vi "process_display_IMAQ_imaq.vi"() -> ()   [LabVIEW 2011, in "Fiberscope_library.lvlib"]
uses:
  Fiberscope_library.lvlib
  typedefs/image_size_I32.ctl
  typedefs/control_process_state_enum.ctl
  typedefs/control_process_state_cluster.ctl
  typedefs/feedback_from_process_enum.ctl
  typedefs/feedback_to_watchdog.ctl
  <vilib>/Analysis/NI_AALBase.lvlib
  <vilib>/vision/Image Controls.llb/IMAQ Image.ctl
  typedefs/element_imaq_images_cluster.ctl
  typedefs/color_palette_enum.ctl
panel:
  in  "Ch1 lower":dbl
  in  "Ch0 lower":dbl
  in  "W2 Ch1 Color":T1=enum."Grayscale"
  in  "W2 Ch0 Color":T1=enum."Grayscale"
  in  "Ch1 upper":dbl
  in  "Ch0 upper":dbl
  out "Ch1 Max":dbl
  out "Ch0 Max":dbl
  in  "W1 Ch1 Color":T1=enum."Grayscale"
  out "Histogram Ch1":T2(graph)
  out "Histogram Ch0":T2(graph)
  out "Window 2":T3(plugin-control)
  out "Window 1":T3(plugin-control)
  in  "Ch1 Full range":bool
  in  "Ch1 Optimize":bool
  in  "W1 Ch0 Color":T1=enum."Grayscale"
  in  "Ch0 Full range":bool
  in  "Ch0 Optimize":bool
  out "Local exit":bool
  out "error out":errorcluster
  in  "error in":errorcluster
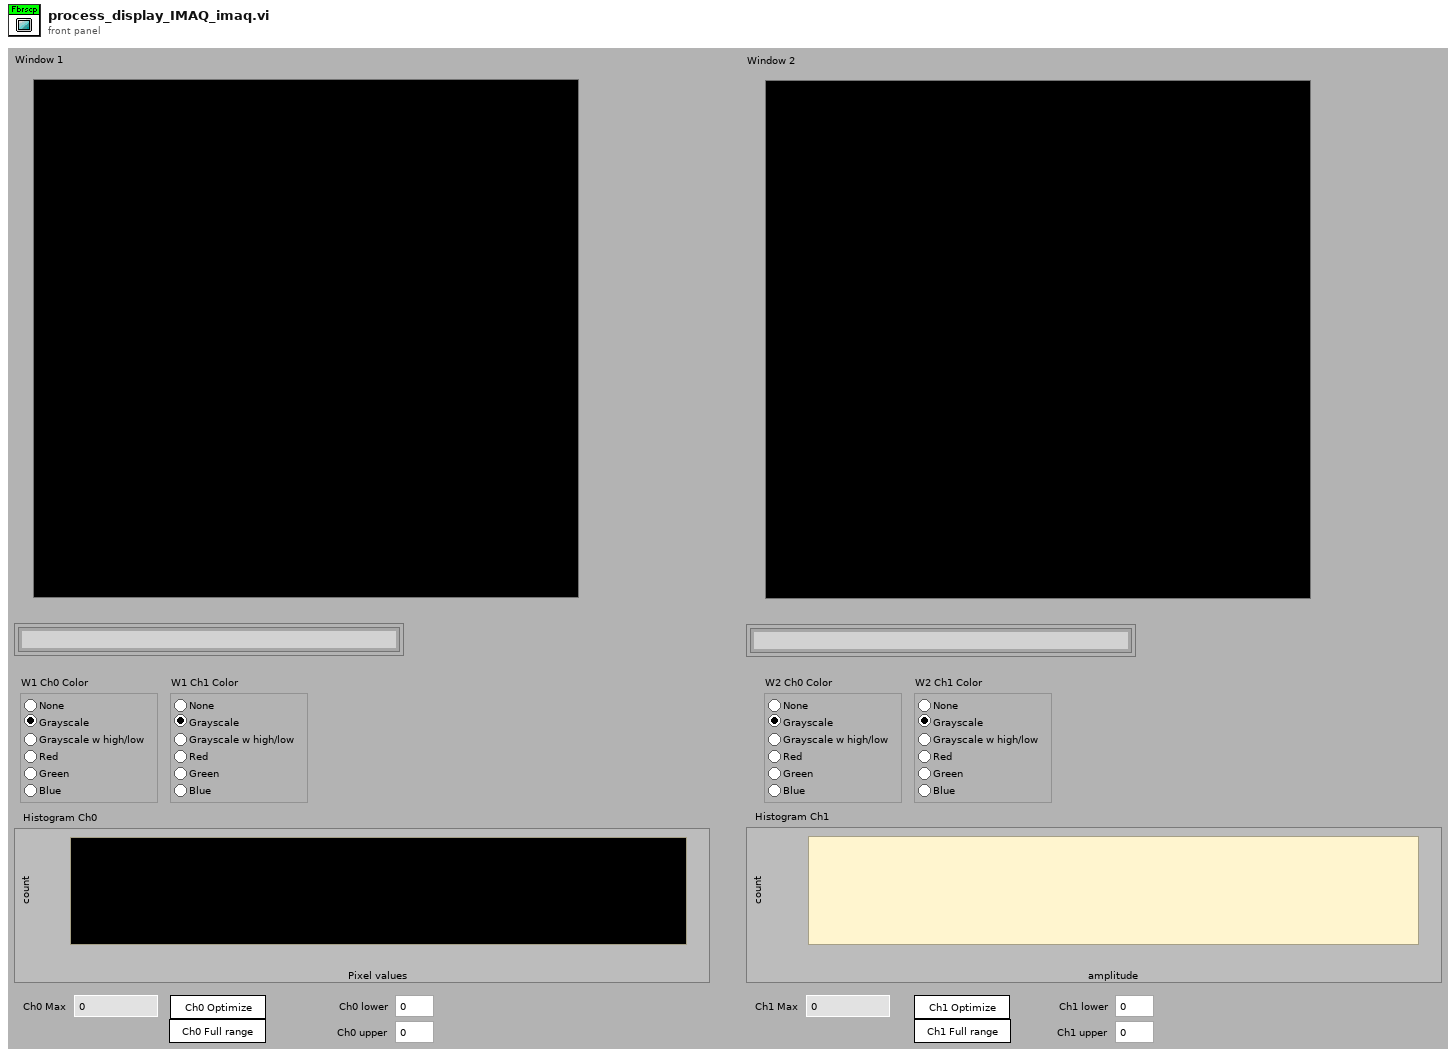
[diagram p1: front panel]
types:
  T1 = typedef "Fiberscope_library.lvlib/color_palette_enum.ctl" = enum32{"None", "Grayscale", "Grayscale w high/low", "Red", "Green", "Blue"}
  T2 = cluster{"X Values":dbl[], "Histogram: h(x)":i32[]}
  T3 = typedef "IMAQ Image.ctl" = refnum<image>
  T4 = typedef "Fiberscope_library.lvlib/element_imaq_images_cluster.ctl" = cluster{"Images":T3[], "#channels":i32, "Last element?":bool}
  T5 = typedef "Fiberscope_library.lvlib/feedback_to_watchdog.ctl" = cluster{"Feedback_from_process_enum":T6, "Process_name":string}
  T6 = typedef "Fiberscope_library.lvlib/feedback_from_process_enum.ctl" = enum16{"Has_initialised", "Changed_parameters", "Has_started", "Has_stopped", "Has_quitted", "Is_running", "Has_finished", "Custom"}
  T7 = typedef "Fiberscope_library.lvlib/control_process_state_cluster.ctl" = cluster{"Control_process_state_enum":T8, "variant":variant}
  T8 = typedef "Fiberscope_library.lvlib/control_process_state_enum.ctl" = enum16{"Init", "Quit", "Start", "Stop", "Change_parameters", "Running", "Finish", "Custom"}
  T9 = typedef "LVCursorListTypeDef.ctl" = cluster{"Name":string, "Color":u32, "Style":u8, "Point Style":u8, "Name Visible":bool, "Allow Drag":bool, "Cursor Mode":u32, "Plot":i32, "Index":i32, "Position":cluster{"X":dbl, "Y":dbl}, "X Scale":u32, "Y Scale":u32, "Watch Plots":i32[], "Watch All Plots":bool, "Plot Area":i32, "Label Offset":cluster{"X":dbl, "Y":dbl}}[]
  T10 = cluster{"Name":string, "Color":u32, "Style":u8, "Point Style":u8, "Name Visible":bool, "Allow Drag":bool, "Cursor Mode":u32, "Plot":i32, "Index":i32, "Position":cluster{"X":dbl, "Y":dbl}, "X Scale":u32, "Y Scale":u32, "Watch Plots":i32[], "Watch All Plots":bool, "Plot Area":i32, "Label Offset":cluster{"X":dbl, "Y":dbl}}
  T11 = typedef "Image Type" = u32
  T12 = typedef "Fiberscope_library.lvlib/image_size_I32.ctl" = i32
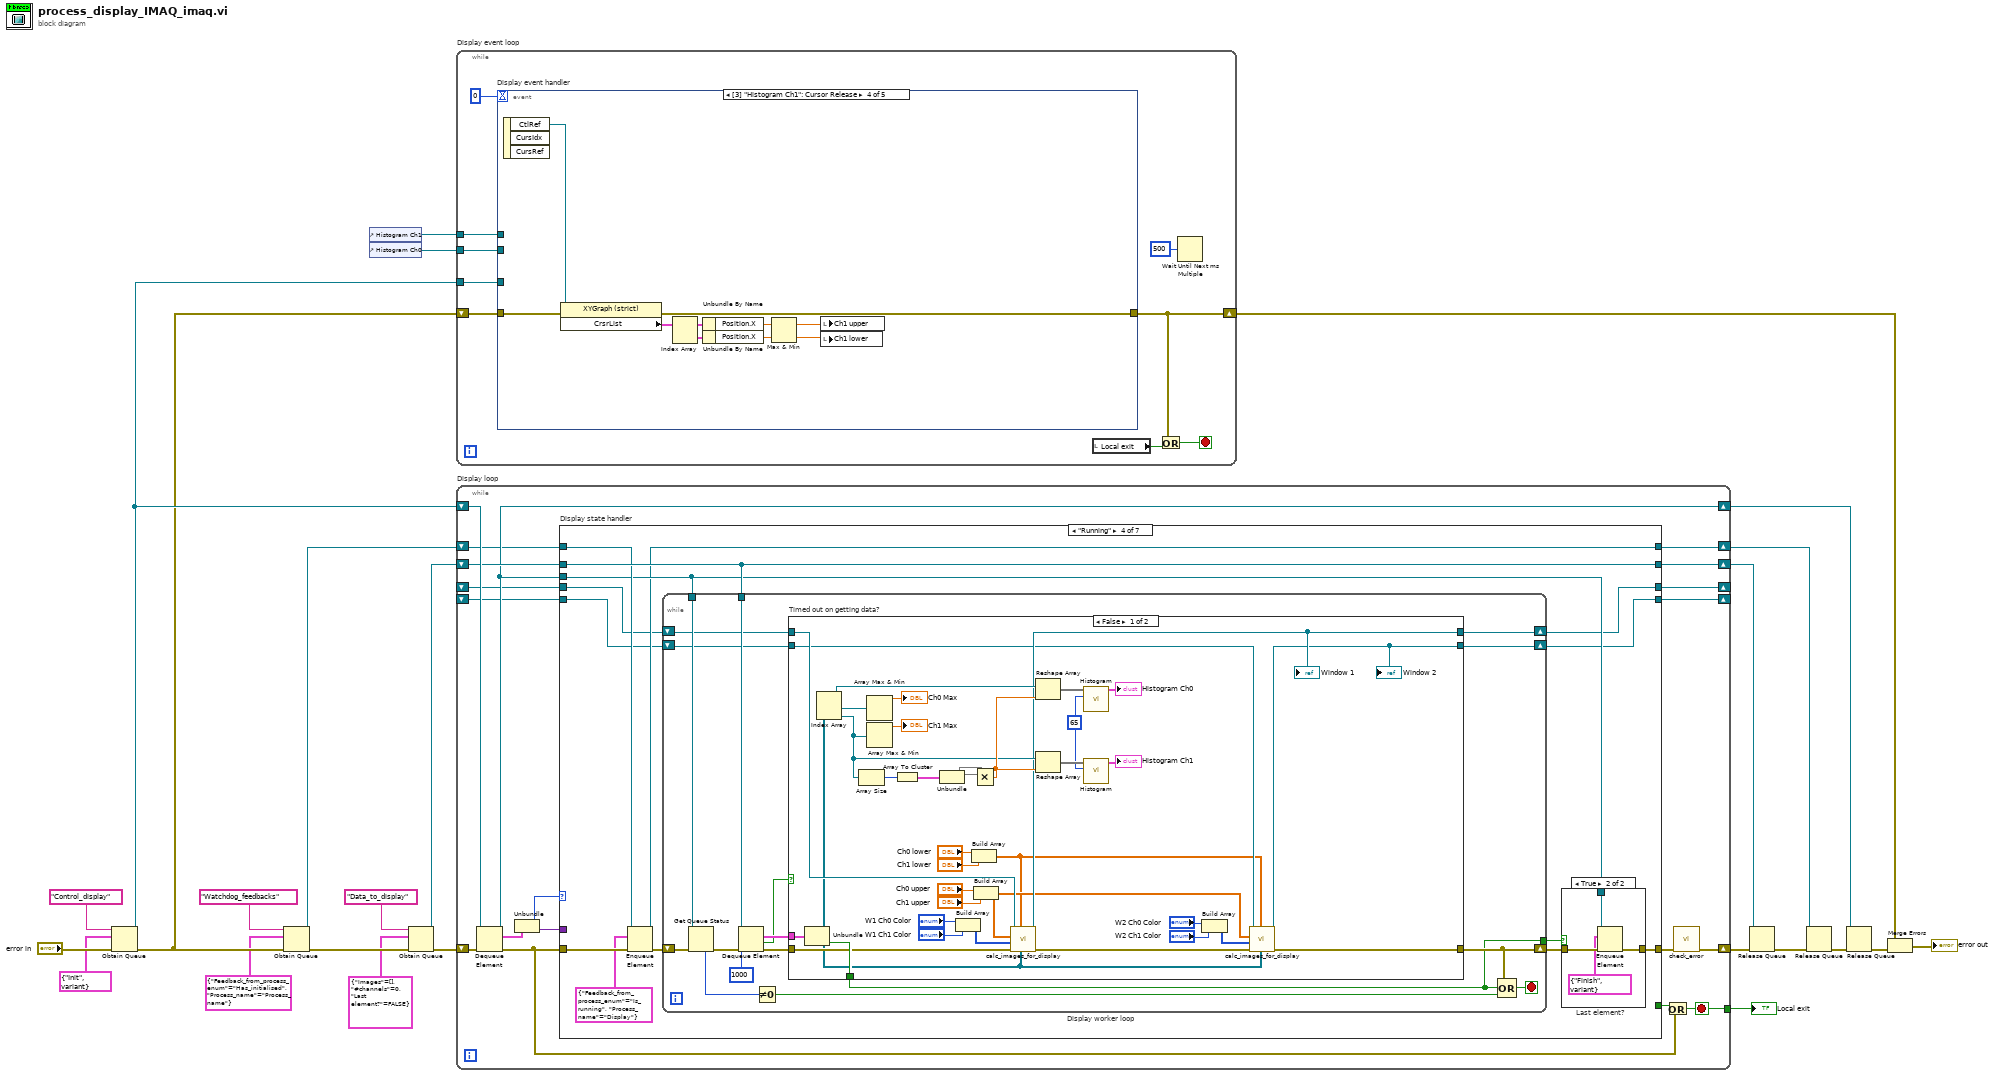
[diagram p0: block diagram]
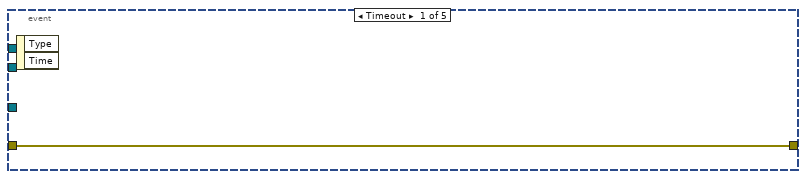
[diagram p2: hidden frame]
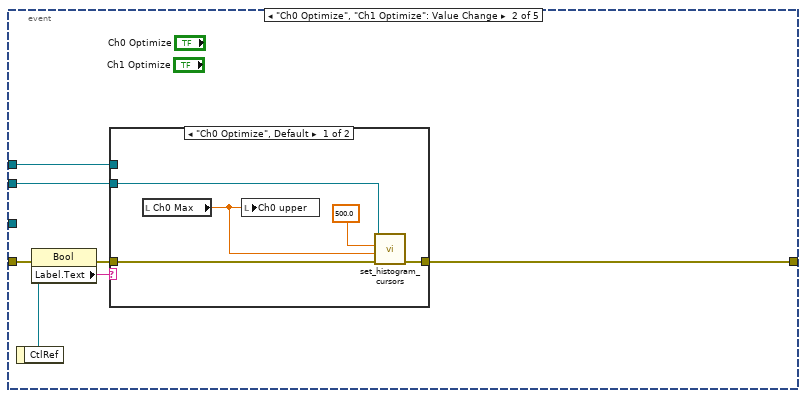
[diagram p3: hidden frame]
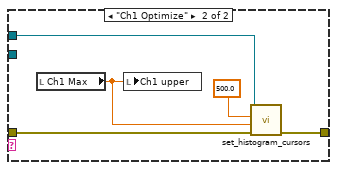
[diagram p4: hidden frame]
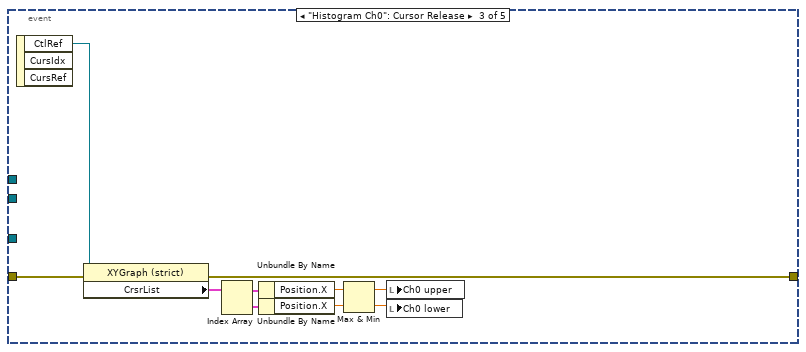
[diagram p5: hidden frame]
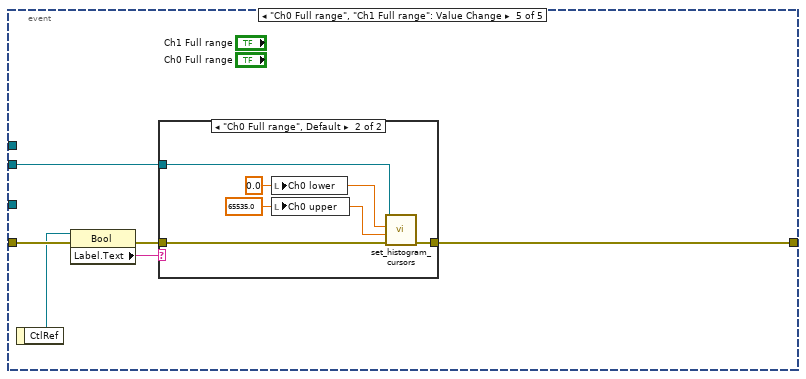
[diagram p6: hidden frame]
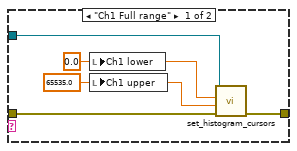
[diagram p7: hidden frame]
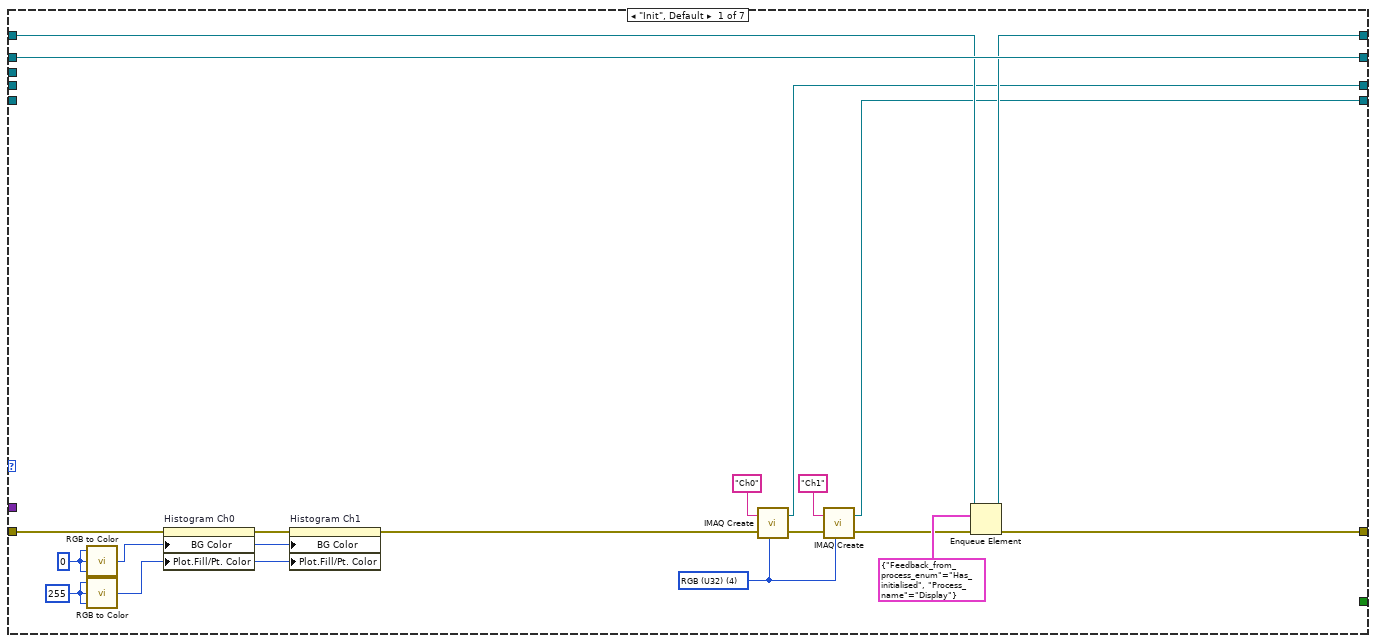
[diagram p8: hidden frame]
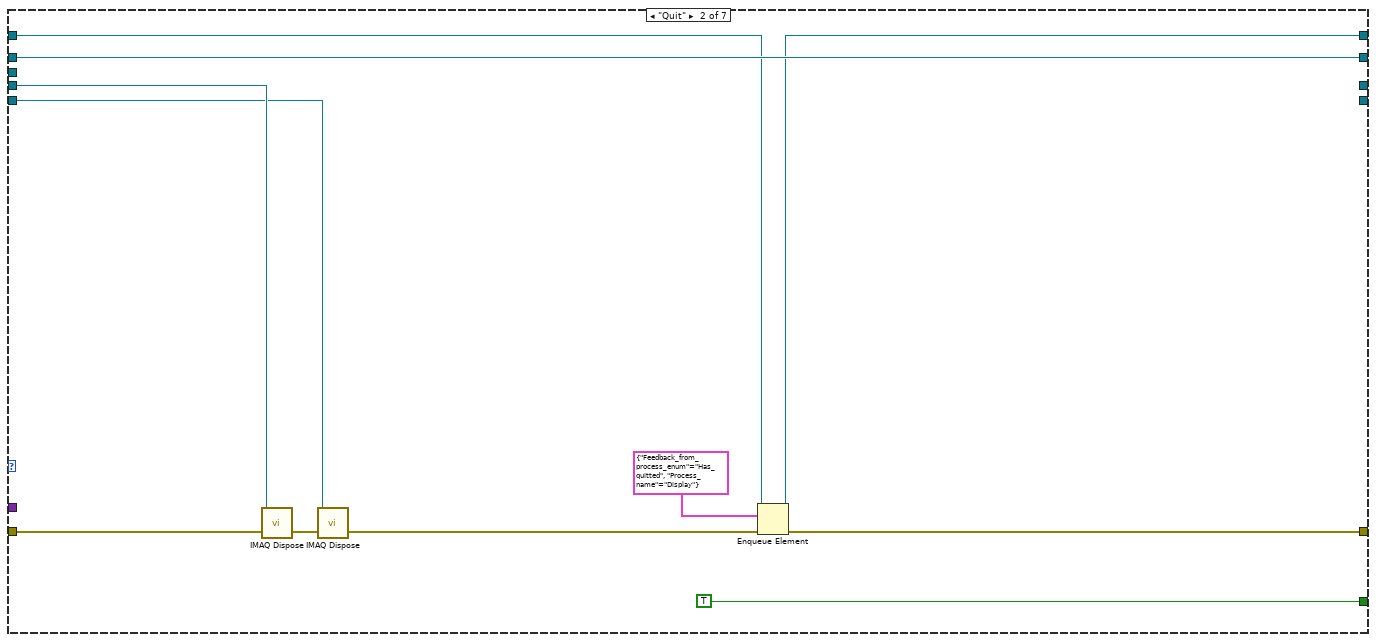
[diagram p9: hidden frame]
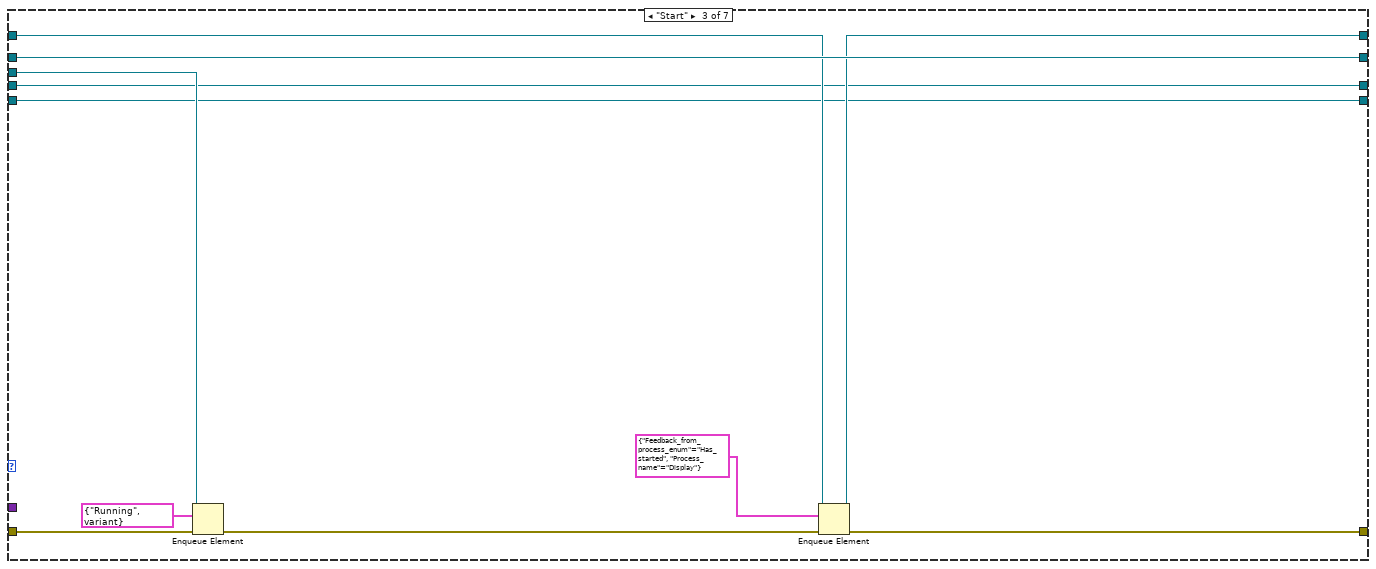
[diagram p10: hidden frame]
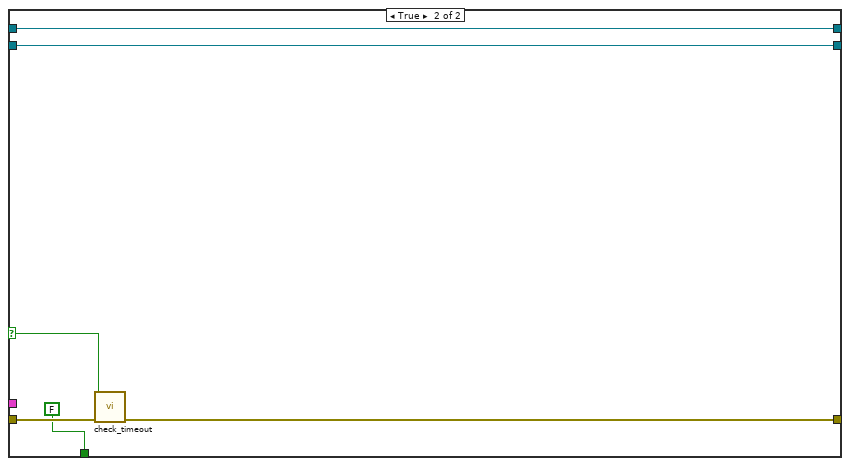
[diagram p12: hidden frame]
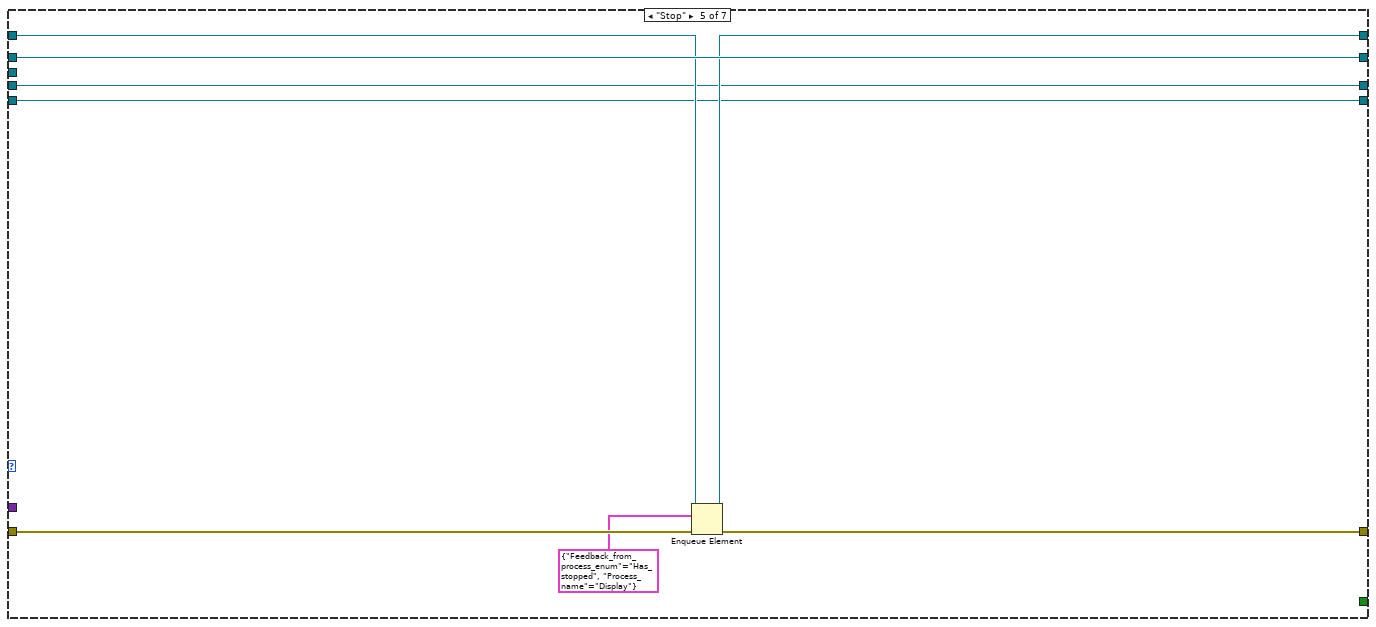
[diagram p13: hidden frame]
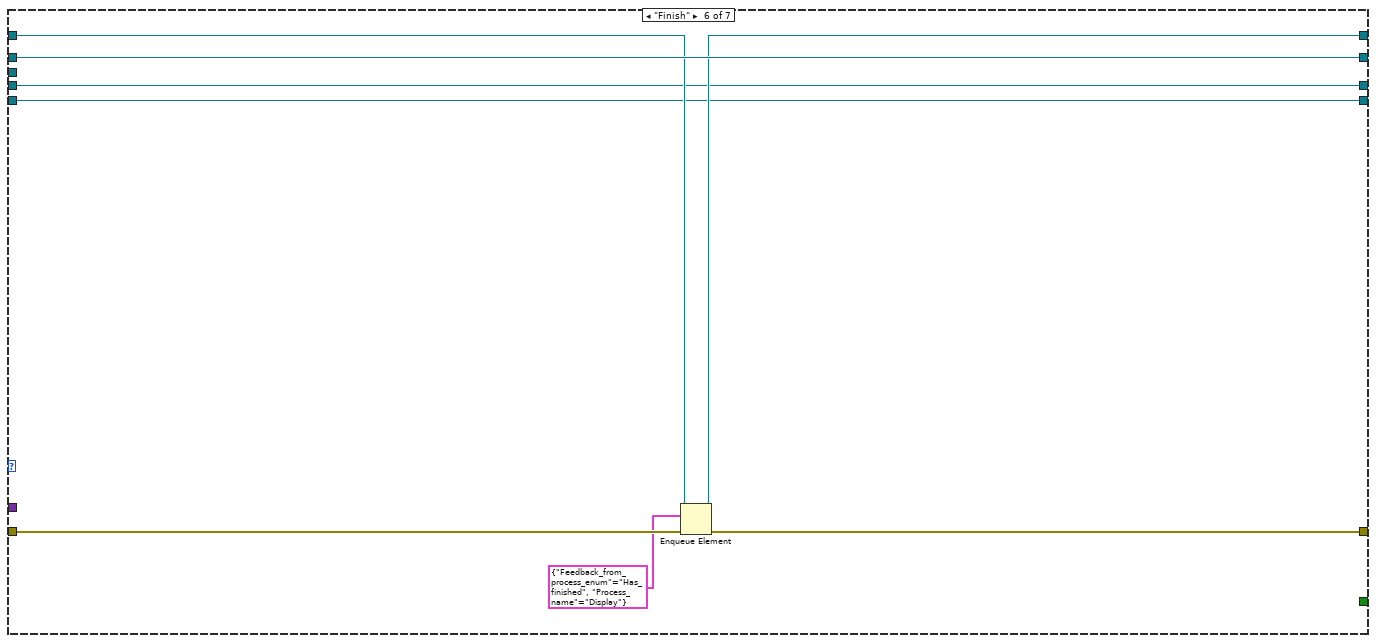
[diagram p14: hidden frame]
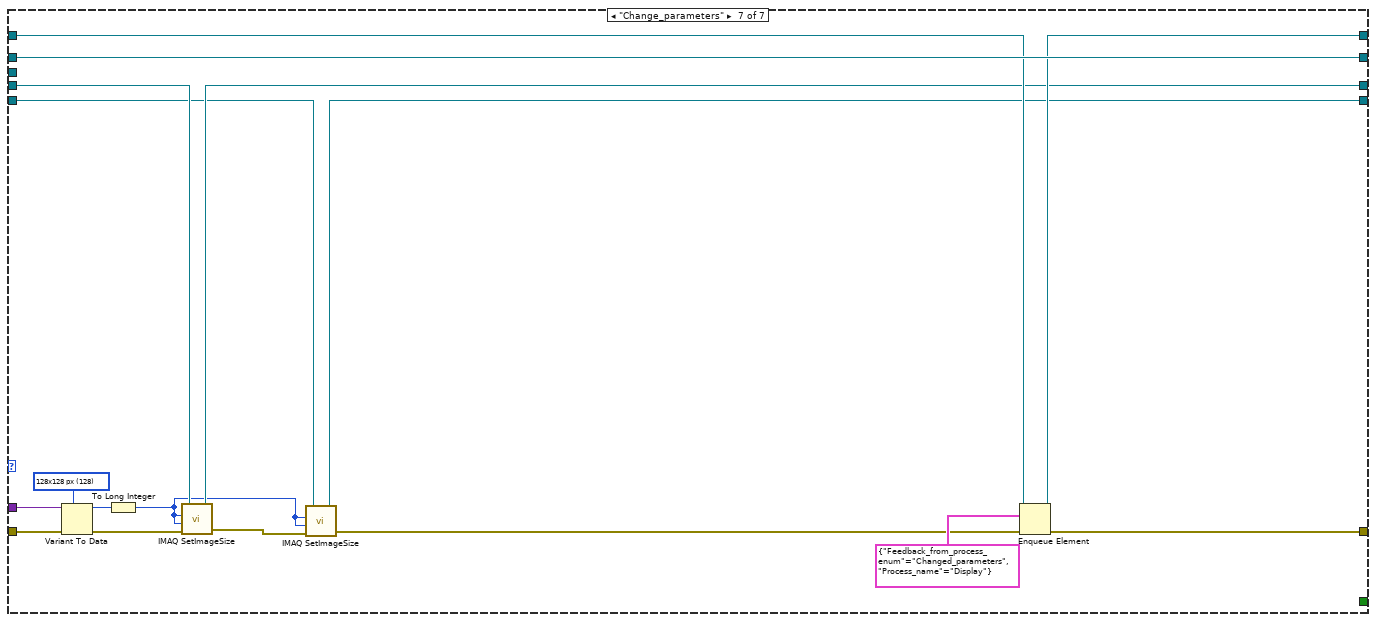
[diagram p15: hidden frame]
diagram:
  n1 = Obtain Queue(name (unnamed)="Control_display", element data type=T7 {"Control_process_state_enum"=enum."Init", "variant"=variant} ("Control_process_state_cluster"), error in (no error)="error in") -> (queue out=w15:refnum<queue>, error out=w10:errorcluster)  [unwired: 2 in, 1 out]
  n2 = Obtain Queue(name (unnamed)="Watchdog_feedbacks", element data type=T5 {"Feedback_from_process_enum"=enum."Has_initialised", "Process_name"="Process_name"}, error in (no error)=w10) -> (queue out=w8:refnum<queue>, error out=w9:errorcluster)  [unwired: 2 in, 1 out]
  n3 = control-ref of="Histogram Ch1"() -> (w3:refnum<vi>)
  n4 = control-ref of="Histogram Ch0"() -> (w2:refnum<vi>)
  n5 = Obtain Queue(name (unnamed)="Data_to_display", element data type=T4 {"Images"=[], "#channels"=0, "Last element?"=FALSE} ("Element_imaq_images_cluster"), error in (no error)=w9) -> (queue out=w19:refnum<queue>, error out=w21:errorcluster)  [unwired: 2 in, 1 out]
  n6 = while "Display event loop" {
    tunnel: w15 -> [w33]
    shift-right: [w28] -> w13
    shift-left: w10 -> [w32]
    tunnel: w3 -> [w27]
    tunnel: w2 -> [w26]
    stop <- w29 stop-if-true
    n7 = event "Display event handler" shown="[3] \"Histogram Ch1\": Cursor Release" {
      selector: _ -> [_ _ _ _ _]
      dyn-events: _ -> [_ _ _ _ _]
      timeout: 0 -> [_ _ _ _ _]
      tunnel: w33 -> [_ _ _ _ _]
      tunnel: w32 -> [w35 w40 w62 w67 w78]
      tunnel: [w35 w38 w61 w66 w74] -> w28
      tunnel: w27 -> [_ w37 _ _ _]
      tunnel: w26 -> [_ w36 _ _ w73]
      event Timeout {
        n8 = event-data() -> ()  [unwired: 1 in, 2 out]
      }
      event "Ch0 Optimize", "Ch1 Optimize": Value Change {
        n9 = event-data() -> ("CtlRef"=w42:refnum<vi>)  [unwired: 1 in]
        n10 = property class="Bool"(reference=w42, error in=w40) -> (error out=w39:errorcluster, "Label.Text"=w41:string)  [unwired: 1 out]
        n11 = case shown="\"Ch0 Optimize\", Default" w41 {
          tunnel: w39 -> [w47 w52]
          tunnel: [w46 w50] -> w38
          tunnel: w37 -> [_ w49]
          tunnel: w36 -> [w45 _]
          frame "Ch0 Optimize", Default {
            n12 = local read "Ch0 Max"() -> (w44:dbl)
            n13 = local write "Ch0 upper"(w44) -> ()
            n14 = call "set_histogram_cursors.vi"("error in (no error)"=w47, "Max pos"=w44, "Min pos"=500.0, "Histogram reference in"=w45) -> ("error out"=w46:errorcluster)  [unwired: 7 in]
          }
          frame "Ch1 Optimize" {
            n15 = local read "Ch1 Max"() -> (w51:dbl)
            n16 = local write "Ch1 upper"(w51) -> ()
            n17 = call "set_histogram_cursors.vi"("error in (no error)"=w52, "Max pos"=w51, "Min pos"=500.0, "Histogram reference in"=w49) -> ("error out"=w50:errorcluster)  [unwired: 7 in]
          }
        }
      }
      event "Histogram Ch0": Cursor Release {
        n18 = event-data() -> ("CtlRef"=w60:refnum<vi>)  [unwired: 1 in, 2 out]
        n19 = property class="XYGraph (strict)"(reference=w60, error in=w62) -> (error out=w61:errorcluster, "CrsrList"=w55:T9)  [unwired: 1 out]
        n20 = Index Array(array=w55) -> (element #1=w59:T10, element #2=w58:T10)  [unwired: 2 in]
        n21 = Unbundle By Name(w59) -> ("Position.X"=w57:dbl)
        n22 = Unbundle By Name(w58) -> ("Position.X"=w56:dbl)
        n23 = Max & Min(x=w57, y=w56) -> (max(x,y)=w54:dbl, min(x,y)=w53:dbl)
        n24 = local write "Ch0 upper"(w54) -> ()
        n25 = local write "Ch0 lower"(w53) -> ()
      }
      event "Histogram Ch1": Cursor Release {
        n26 = event-data() -> ("CtlRef"=w65:refnum<vi>)  [unwired: 1 in, 2 out]
        n27 = property class="XYGraph (strict)"(reference=w65, error in=w67) -> (error out=w66:errorcluster, "CrsrList"=w68:T9)  [unwired: 1 out]
        n28 = Index Array(array=w68) -> (element #1=w72:T10, element #2=w71:T10)  [unwired: 2 in]
        n29 = Unbundle By Name(w72) -> ("Position.X"=w70:dbl)
        n30 = Unbundle By Name(w71) -> ("Position.X"=w69:dbl)
        n31 = Max & Min(x=w70, y=w69) -> (max(x,y)=w64:dbl, min(x,y)=w63:dbl)
        n32 = local write "Ch1 upper"(w64) -> ()
        n33 = local write "Ch1 lower"(w63) -> ()
      }
      event "Ch0 Full range", "Ch1 Full range": Value Change {
        n34 = event-data() -> ("CtlRef"=w77:refnum<vi>)  [unwired: 1 in]
        n35 = property class="Bool"(reference=w77, error in=w78) -> (error out=w75:errorcluster, "Label.Text"=w76:string)  [unwired: 1 out]
        n36 = case shown="\"Ch0 Full range\", Default" w76 {
          tunnel: w75 -> [w83 w88]
          tunnel: [w82 w87] -> w74
          tunnel: w73 -> [w81 w86]
          frame "Ch1 Full range" {
            w80 = 0.0 ("Ch1 lower")
            w79 = 65535.0 ("Ch1 scaler")
            n37 = local write "Ch1 lower"(w80) -> ()
            n38 = local write "Ch1 upper"(w79) -> ()
            n39 = call "set_histogram_cursors.vi"("error in (no error)"=w83, "Max pos"=w79, "Min pos"=w80, "Histogram reference in"=w81) -> ("error out"=w82:errorcluster)  [unwired: 7 in]
          }
          frame "Ch0 Full range", Default {
            w85 = 0.0 ("Ch0 lower")
            w84 = 65535.0 ("Ch0 scaler")
            n40 = local write "Ch0 lower"(w85) -> ()
            n41 = local write "Ch0 upper"(w84) -> ()
            n42 = call "set_histogram_cursors.vi"("error in (no error)"=w88, "Max pos"=w84, "Min pos"=w85, "Histogram reference in"=w86) -> ("error out"=w87:errorcluster)  [unwired: 7 in]
          }
        }
      }
    }
    n43 = local read "Local exit"() -> (w30:bool)
    n44 = Or(x=w28, y=w30) -> (x .or. y?=w29:bool)
    n45 = Wait Until Next ms Multiple(millisecond multiple=u32 500) -> ()  [unwired: 1 out]
  }
  n46 = while "Display loop" {
    shift-right: [w101] -> w18
    shift-left: w21 -> [w107]
    shift-right: [w98] -> w23
    shift-left: w15 -> [w106]
    shift-right: [w99] -> w17
    shift-left: w19 -> [w100]
    tunnel: [w97] -> w16
    shift-right: [w93] -> w5
    shift-left: w8 -> [w94]
    shift-right: [w92] -> _
    shift-left: _ -> [w90]
    shift-right: [w91] -> _
    shift-left: _ -> [w89]
    stop <- w97 stop-if-true
    n47 = Dequeue Element(queue=w106, error in (no error)=w107) -> (queue out=w98:refnum<queue>, element=w105:T7, error out=w95:errorcluster)  [unwired: 1 in, 1 out]
    n48 = Unbundle(w105) -> ("Control_process_state_enum"=w103:T8, "variant"=w104:variant)
    n49 = case "Display state handler" shown="\"Running\"" w103 {
      tunnel: w95 -> [w114 w130 w145 w161 w233 w241 w258]
      tunnel: [w125 w135 w147 w157 w232 w240 w256] -> w102
      tunnel: w104 -> [_ _ _ _ _ _ w257]
      tunnel: w100 -> [w126 w137 w148 w162 w234 w242 w259]
      tunnel: [w126 w137 w148 w162 w234 w242 w259] -> w99
      tunnel: w98 -> [_ _ w143 w156 _ _ _]
      tunnel: [_ TRUE _ _ _ _ _] -> w96
      tunnel: w94 -> [w124 w134 w146 w159 w231 w239 w255]
      tunnel: [w123 w133 w141 w154 w230 w238 w253] -> w93
      tunnel: [w116 _ w139 w150 w228 w236 w247] -> w92
      tunnel: [w115 _ w138 w149 w227 w235 w245] -> w91
      tunnel: w90 -> [_ w128 w139 w151 w228 w236 w248]
      tunnel: w89 -> [_ w127 w138 w152 w227 w235 w246]
      frame "Init", Default {
        w112 = u8 0 ("R")
        w113 = u8 255 ("R")
        w118 = T11 4 items=["Grayscale (U8)", "Grayscale (I16)", "Grayscale (SGL)", "Complex (CSG)", "RGB (U32)", "HSL (U32)", "RGB (U64)", "Grayscale (U16)"] ("Image Type")
        n50 = call <vilib>:"RGB to Color.vi"("B"=w112, "G"=w112, "R"=w112) -> ("Color"=w109:u32)
        n51 = call <vilib>:"RGB to Color.vi"("B"=w113, "G"=w113, "R"=w113) -> ("Color"=w108:u32)
        n52 = property on="Histogram Ch0" class="XYGraph (strict)"(error in=w114, "BG Color"=w109, "Plot.Fill/Pt. Color"=w108) -> (error out=w111:errorcluster)  [unwired: 1 in, 1 out]
        n53 = property on="Histogram Ch1" class="XYGraph (strict)"(error in=w111, "BG Color"=w109, "Plot.Fill/Pt. Color"=w108) -> (error out=w110:errorcluster)  [unwired: 1 in, 1 out]
        n54 = call "IMAQ Create"("Image Name"="Ch0", "Image Type"=w118, "error in (no error)"=w110) -> ("New Image"=w116:T3, "error out"=w121:errorcluster)  [unwired: 2 in]
        n55 = call "IMAQ Create"("Image Name"="Ch1", "Image Type"=w118, "error in (no error)"=w121) -> ("New Image"=w115:T3, "error out"=w117:errorcluster)  [unwired: 2 in]
        n56 = Enqueue Element(queue=w124, element=T5 {"Feedback_from_process_enum"=enum."Has_initialised", "Process_name"="Display"}, error in (no error)=w117) -> (queue out=w123:refnum<queue>, error out=w125:errorcluster)  [unwired: 1 in, 1 out]
      }
      frame "Quit" {
        n57 = call "IMAQ Dispose"("Image"=w128, "error in (no error)"=w130) -> ("error out"=w131:errorcluster)  [unwired: 4 in]
        n58 = call "IMAQ Dispose"("Image"=w127, "error in (no error)"=w131) -> ("error out"=w129:errorcluster)  [unwired: 4 in]
        n59 = Enqueue Element(queue=w134, element=T5 {"Feedback_from_process_enum"=enum."Has_quitted", "Process_name"="Display"}, error in (no error)=w129) -> (queue out=w133:refnum<queue>, error out=w135:errorcluster)  [unwired: 1 in, 1 out]
      }
      frame "Start" {
        n60 = Enqueue Element(queue=w143, element=T7 {"Control_process_state_enum"=enum."Running", "variant"=variant} ("Control_process_state_cluster"), error in (no error)=w145) -> (error out=w144:errorcluster)  [unwired: 1 in, 2 out]
        n61 = Enqueue Element(queue=w146, element=T5 {"Feedback_from_process_enum"=enum."Has_started", "Process_name"="Display"}, error in (no error)=w144) -> (queue out=w141:refnum<queue>, error out=w147:errorcluster)  [unwired: 1 in, 1 out]
      }
      frame "Running" {
        n62 = Enqueue Element(queue=w159, element=T5 {"Feedback_from_process_enum"=enum."Is_running", "Process_name"="Display"}, error in (no error)=w161) -> (queue out=w154:refnum<queue>, error out=w160:errorcluster)  [unwired: 1 in, 1 out]
        n63 = while "Display worker loop" {
          tunnel: w156 -> [w183]
          tunnel: w162 -> [w180]
          shift-right: [w173] -> w158
          shift-left: w160 -> [w184]
          tunnel: [w172] -> w155
          shift-right: [w169] -> w149
          shift-left: w152 -> [w171]
          shift-right: [w168] -> w150
          shift-left: w151 -> [w170]
          stop <- w178 stop-if-true
          n64 = Get Queue Status(queue=w183, error in (no error)=w184) -> (error out=w181:errorcluster, # elements in queue=w182:i32)  [unwired: 1 in, 6 out]
          n65 = Dequeue Element(queue=w180, timeout in ms (-1)=1000, error in (no error)=w181) -> (element=w177:T4, timed out?=w174:bool, error out=w176:errorcluster)  [unwired: 1 out]
          n66 = Not Equal To 0?(x=w182) -> (x != 0?=w179:bool)
          n67 = case "Timed out on getting data?" shown="False" w174 {
            selector: w174 -> [_ w224]
            tunnel: w177 -> [w220 _]
            tunnel: w176 -> [w204 w226]
            tunnel: [w193 w225] -> w173
            tunnel: [w219 FALSE ("Last element?")] -> w172
            tunnel: w171 -> [w189 w222]
            tunnel: w170 -> [w198 w221]
            tunnel: [w188 w222] -> w169
            tunnel: [w192 w221] -> w168
            frame False {
              w210 = 65 ("intervals")
              n68 = Unbundle(w220) -> ("Images"=w191:T3[], "Last element?"=w219:bool)  [unwired: 1 out]
              n69 = Index Array(array=w191) -> (element #1=w208:T3, element #2=w207:T3)  [unwired: 2 in]
              n70 = Array Size(array=w207) -> (size(s)=w214:i32)
              n71 = Array Max & Min(array=w208) -> (max value=→"Ch0 Max":dbl)  [unwired: 3 out]
              n72 = Array Max & Min(array=w207) -> (max value=→"Ch1 Max":dbl)  [unwired: 3 out]
              n73 = Array To Cluster(array=w214) -> (cluster=w215:cluster{"[0]":void, "[1]":void})
              n74 = Unbundle(w215) -> ("[0]"=w216, "[1]"=w217)
              n75 = Build Array("W1 Ch0 Color", "W1 Ch1 Color") -> (w201:T1[])
              n76 = Build Array("Ch0 lower", "Ch1 lower") -> (w185:dbl[])
              n77 = Multiply(x=w216, y=w217) -> (x*y=w212:dbl)
              n78 = Build Array("Ch0 upper", "Ch1 upper") -> (w190:dbl[])
              n79 = call "calc_images_for_display.vi"("Raw data in"=w191, "Lower bounds array"=w185, "error in"=w204, "Color tables display"=w201, "Upper bounds array"=w190, "Image in"=w198) -> ("error out"=w197:errorcluster, "Image Out"=w192:T3)  [unwired: 4 in]
              "Window 1" <- w192
              n80 = Reshape Array(w208, w212) -> (w213:void[])
              n81 = Reshape Array(w207, w212) -> (w211:void[])
              n82 = call <vilib>:"Histogram.vi"("intervals"=w210, "X"=w213) -> ("Histogram Graph"=→"Histogram Ch0":T2)  [unwired: 6 in, 3 out]
              n83 = call <vilib>:"Histogram.vi"("intervals"=w210, "X"=w211) -> ("Histogram Graph"=→"Histogram Ch1":T2)  [unwired: 6 in, 3 out]
              n84 = Build Array("W2 Ch0 Color", "W2 Ch1 Color") -> (w194:T1[])
              n85 = call "calc_images_for_display.vi"("Raw data in"=w191, "Lower bounds array"=w185, "error in"=w197, "Color tables display"=w194, "Upper bounds array"=w190, "Image in"=w189) -> ("error out"=w193:errorcluster, "Image Out"=w188:T3)  [unwired: 4 in]
              "Window 2" <- w188
            }
            frame True {
              n86 = call "check_timeout.vi"("error in"=w226, "Timeout?"=w224) -> ("error out"=w225:errorcluster)  [unwired: 9 in]
            }
          }
          n87 = Compound Arithmetic op=OR(w173, w172, w179) -> (w178:bool)
        }
        n88 = case "Last element?" shown="True" w155 {
          tunnel: w158 -> [w163 w167]
          tunnel: [w163 w166] -> w157
          tunnel: w156 -> [_ w165]
          frame False {
          }
          frame True {
            n89 = Enqueue Element(queue=w165, element=T7 {"Control_process_state_enum"=enum."Finish", "variant"=variant} ("Control_process_state_cluster"), error in (no error)=w167) -> (error out=w166:errorcluster)  [unwired: 1 in, 2 out]
          }
        }
      }
      frame "Stop" {
        n90 = Enqueue Element(queue=w231, element=T5 {"Feedback_from_process_enum"=enum."Has_stopped", "Process_name"="Display"}, error in (no error)=w233) -> (queue out=w230:refnum<queue>, error out=w232:errorcluster)  [unwired: 1 in, 1 out]
      }
      frame "Finish" {
        n91 = Enqueue Element(queue=w239, element=T5 {"Feedback_from_process_enum"=enum."Has_finished", "Process_name"="Display"}, error in (no error)=w241) -> (queue out=w238:refnum<queue>, error out=w240:errorcluster)  [unwired: 1 in, 1 out]
      }
      frame "Change_parameters" {
        w254 = T12 128 items=["128x128 px"=128, "256x256 px"=256, "512x512 px"=512] ("Image size")
        n92 = Variant To Data(error in=w258, type=w254, Variant=w257) -> (data=w244:T12, error out=w250:errorcluster)
        n93 = To Long Integer(number=w244) -> (32bit integer=w243:T12)
        n94 = call "IMAQ SetImageSize"("error in (no error)"=w250, "Y Resolution"=w243, "X Resolution"=w243, "Image"=w248) -> ("error out"=w251:errorcluster, "Image Out"=w247:T3)  [unwired: 1 in]
        n95 = call "IMAQ SetImageSize"("error in (no error)"=w251, "Y Resolution"=w243, "X Resolution"=w243, "Image"=w246) -> ("error out"=w249:errorcluster, "Image Out"=w245:T3)  [unwired: 1 in]
        n96 = Enqueue Element(queue=w255, element=T5 {"Feedback_from_process_enum"=enum."Changed_parameters", "Process_name"="Display"}, error in (no error)=w249) -> (queue out=w253:refnum<queue>, error out=w256:errorcluster)  [unwired: 1 in, 1 out]
      }
    }
    n97 = Or(x=w96, y=w95) -> (x .or. y?=w97:bool)
    n98 = call "check_error.vi"("error in"=w102) -> ("error out"=w101:errorcluster)  [unwired: 10 in]
  }
  "Local exit" <- w16
  n99 = Release Queue(queue=w17, error in (no error)=w18) -> (error out=w7:errorcluster)  [unwired: 1 in, 2 out]
  n100 = Release Queue(queue=w5, error in (no error)=w7) -> (error out=w6:errorcluster)  [unwired: 1 in, 2 out]
  n101 = Release Queue(queue=w23, error in (no error)=w6) -> (error out=w14:errorcluster)  [unwired: 1 in, 2 out]
  n102 = Merge Errors(w13, w14) -> (→"error out":errorcluster)
